vi "Test Geometry.vi"() -> ()   [LabVIEW 2011]
uses:
  gvision/gVisionSource/Release/gVision.dll
panel:
  out "return type":string
  in  "path":path
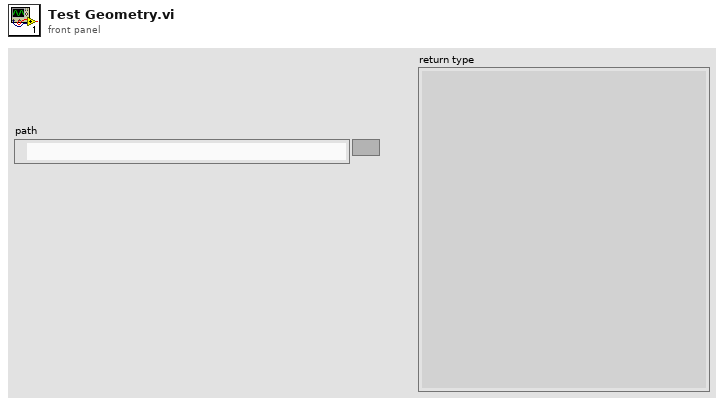
[diagram p1: front panel]
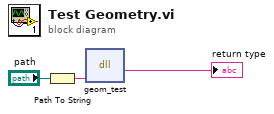
[diagram p0: block diagram]
diagram:
  n1 = Path To String(path="path") -> (string=w2:string)
  n2 = dll-call lib="C:/Users/husker/Desktop/gvision/gVisionSource/Release/gVision.dll" fn="geom_test"("arg1"=w2) -> ("return type"=→"return type":string)  [unwired: 4 in, 2 out]
